vi "Actor Core.vi"(8 "error in":errorcluster, 11 "Line Tracker in":refnum<class "Line Tracker.lvclass">) -> (0 "error out":errorcluster, 3 "Actor out":refnum<class "Actor.lvclass">)   [LabVIEW 2026, in "Line Tracker.lvlib" / "Line Tracker.lvclass"]
doc: "<p>(<strong>Filename</strong>: <span class=\"dnl\">Actor Framework.lvlib:Actor.lvclass:Actor Core.vi</span>)</p>\n<p>Receives messages to the actor, reacts to them, and initiates any error handling that may shut the actor down.</p>\n<p>Descendant classes may override this VI to append parallel tasks for the actor to complete while it handles messages. Overrides use the <a href=\"nihelplauncher://docs/csh?context=lvcore_glang_udclass\">Call Parent Class Method</a> node.</p>"
uses:
  Line Tracker.lvclass
  <vilib>/ActorFramework/Actor/Actor.lvclass
  Line Tracker.lvclass/Line Tracker.ctl
  Tracking Values.ctl
  CTI-Grove/Examples/Sourcecode/cti-drivers-lv-visa-simple/Examples/Driver/CTIPicoVISA.lvlib
  3af2abc0-a50f-3fe3-70cf-f76fd197d63f.vi
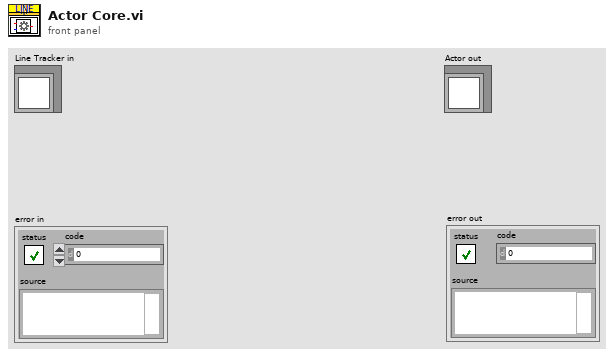
[diagram p1: front panel]
types:
  T1 = typedef "Tracking Values.ctl" = cluster{"LEFT":bool, "CENTRE":bool, "RIGHT":bool}
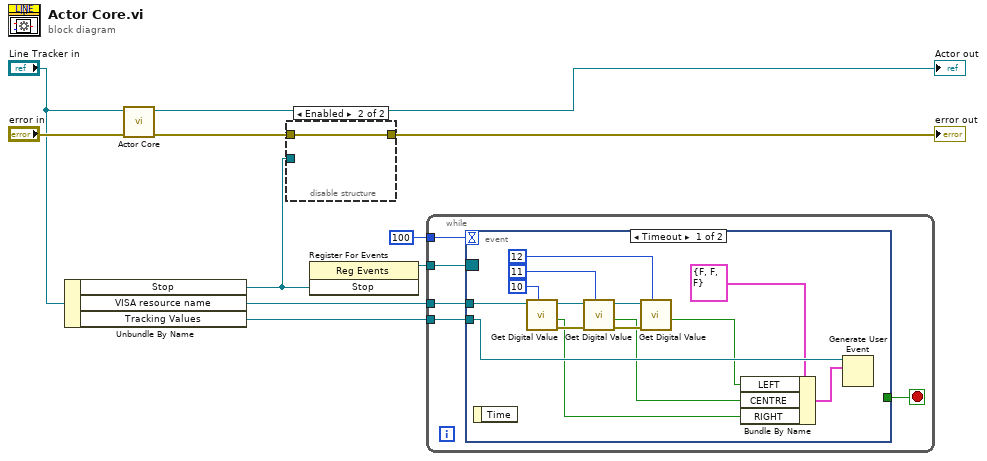
[diagram p0: block diagram]
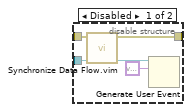
[diagram p2: hidden frame]
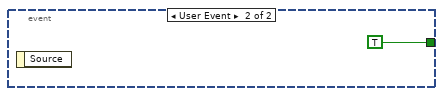
[diagram p3: hidden frame]
diagram:
  n1 = Unbundle By Name("Line Tracker in") -> ("Stop"=w1:refnum<user-event>, "VISA resource name"=w6:refnum<visa-resource-name>, "Tracking Values"=w7:refnum<user-event>)
  n2 = call-parent "Actor Core.vi"("error in"="error in", "Actor in"="Line Tracker in") -> ("error out"=w3:errorcluster, "Actor out"=→"Actor out":refnum<class "Actor.lvclass">)  [unwired: 8 in]
  n3 = disable-structure shown="Enabled" {
    disable-tunnel: w3 -> [w15 w16]
    disable-tunnel: [w14 w16] -> w2
    disable-tunnel: w1 -> [w13 _]
    frame Disabled {
      n4 = call "Synchronize Data Flow.vim"("input 4"=w13, "input 1"=w15) -> ("output 4"=w12:refnum<user-event>, "output 1"=w14:errorcluster)  [unwired: 2 in, 2 out]
      n5 = Generate User Event(user event=w12, event data cluster=variant ("event data")) -> ()  [unwired: 2 in, 2 out]
    }
    frame Enabled {
    }
  }
  "error out" <- w2
  n6 = register-events(w1) -> (reference out=w5:refnum<event-registration>)  [unwired: 2 in, 1 out]
  n7 = while {
    tunnel: w7 -> [w18]
    tunnel: w6 -> [w21]
    tunnel: w5 -> [w20]
    tunnel: 100 -> [w19]
    stop <- w17 stop-if-true
    n8 = event shown="[0] Timeout" {
      selector: w20 -> [_ _]
      dyn-events: _ -> [_ _]
      timeout: w19 -> [_ _]
      tunnel: w21 -> [w35 _]
      tunnel: w18 -> [w27 _]
      tunnel: [_ TRUE] -> w17
      event Timeout {
        n9 = event-data() -> ()  [unwired: 1 in, 1 out]
        n10 = call "Get Digital Value.vi"("GPIO"=10, "VISA resource name in"=w35) -> ("error out"=w34:errorcluster, "Value"=w22:bool, "VISA resource name"=w33:refnum<visa-resource-name>)  [unwired: 7 in]
        n11 = call "Get Digital Value.vi"("GPIO"=11, "error in (no error)"=w34, "VISA resource name in"=w33) -> ("error out"=w31:errorcluster, "Value"=w23:bool, "VISA resource name"=w32:refnum<visa-resource-name>)  [unwired: 6 in]
        n12 = call "Get Digital Value.vi"("GPIO"=12, "error in (no error)"=w31, "VISA resource name in"=w32) -> ("Value"=w24:bool)  [unwired: 6 in, 2 out]
        n13 = Bundle By Name(cluster=T1 {"LEFT"=FALSE, "CENTRE"=FALSE, "RIGHT"=FALSE} ("event data"), "LEFT"=w24, "CENTRE"=w23, "RIGHT"=w22) -> (w25:T1)
        n14 = Generate User Event(user event=w27, event data cluster=w25) -> ()  [unwired: 2 in, 2 out]
      }
      event User Event {
        n15 = event-data() -> ()  [unwired: 1 in, 1 out]
      }
    }
  }
